vi "read sim data.vi"(11 "Array IN":u16[][](array[numeric])=array480x764[366720 elements]) -> (3 "Array Out":u16[][](array[numeric]))   [LabVIEW 2022 SP3, in "Sim Camera Driver.lvclass"]
uses:
  Sim Camera Driver.lvclass
  <vilib>/numeric/Random Number (Range) U64.vi
  <vilib>/numeric/sub_Random U32.vi
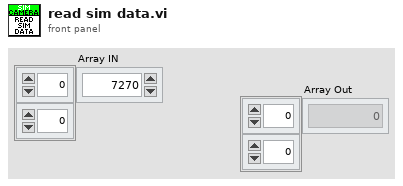
[diagram p1: front panel]
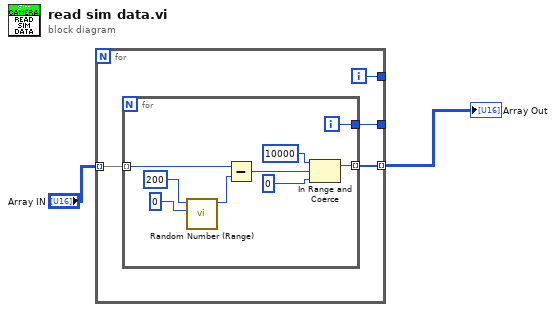
[diagram p0: block diagram]
diagram:
  n1 = for {
    tunnel: [w6] -> w2 mode=indexing
    tunnel: [w5] -> _
    tunnel: [w4] -> _
    tunnel: "Array IN" -> [w3] mode=indexing
    i -> [w5]
    n2 = for {
      tunnel: [w9] -> w6 mode=indexing
      tunnel: [w8] -> w4
      tunnel: w3 -> [w7] mode=indexing
      i -> [w8]
      n3 = call-poly <vilib>:"Random Number (Range).vi"("lower bound (0)"=u16 0, "upper bound (100)"=u16 200) -> ("number"=w15:u64)  [unwired: 9 in]
      n4 = Subtract(x=w7, y=w15) -> (x-y=w12:u64)
      n5 = In Range and Coerce(upper limit=u16 10000, x=w12, lower limit=u16 0) -> (coerced(x)=w9:u64)  [unwired: 1 out]
    }
  }
  "Array Out" <- w2
